vi "lerealtime.vi"() -> ()   [LabVIEW 2016]
uses:
  <vilib>/rvi/interface/nirviOpenFPGA/nirviOpenFPGA.xnode
  <vilib>/rvi/interface/nirviReadWriteControl/nirviReadWriteControl.xnode
  le fpga/le fpga.vi
  NiFpgaLv.dll
  <vilib>/Utility/error.llb/Error Cluster From Error Code.vi
  <vilib>/rvi/errors/niLvFpgaAdjustHostInterfaceError.vi
  FPGA Bitfiles/Controlsoftware2_FPGATarget2_lefpga_X2lKp2O+XjE.lvbitx
  <vilib>/FPGAPlugInAG/cRIO-9074/niLvFpga_Open_cRIO-9074.vi
panel:
  in  "Numeric value out":dbl
  in  "Tab Control":enum32{"Control", "Junk"}(tab)
  out "LE Einzel":dbl
  out "le waist einzel I":fxp<+/-,26,5> format="%.3g"
  out "le Waist Einzel V":fxp<+/-,26,5> format="%.3g"
  out "le waist Y-I":fxp<+/-,26,5> format="%.3g"
  out "le waist Y-V":fxp<+/-,26,5> format="%.3g"
  out "le waist Y+I":fxp<+/-,26,5> format="%.3g"
  out "le waist Y+ V":fxp<+/-,26,5> format="%.3g"
  out "le waist X-I":fxp<+/-,26,5> format="%.3g"
  out "le waist X- V":fxp<+/-,26,5> format="%.3g"
  out "le waist X+ I":fxp<+/-,26,5> format="%.3g"
  out "le waist X+ V":fxp<+/-,26,5> format="%.3g"
  out "le waist Y Steerer -":dbl
  out "le waist Y Steerer +":dbl
  out "le waistX Steerer -":dbl
  out "le waist X Steerer +":dbl
  out "Tank entrance Cryo pump":T1
  out "atten":bool
  out "LE waist fc":bool
  out "LE waist apt":bool
  out "inj image ap":bool
  out "tank entrance fc":bool
  out "Tank Entrance Ion gauge Cluster":T2
  out "LE Waist Ion gauge Cluster 2":T2
  out "Y Steerer -":dbl
  out "Y Steerer +":dbl
  out "X Steerer -":dbl
  out "X Steerer +":dbl
  out "Y Steerer -  2":dbl
  out "Y Steerer +  2":dbl
  in  "X Steerer - 2":dbl
  in  "X Steerer + 2":dbl
  out "Y-I 2":fxp<+/-,26,5> format="%.3g"
  out "Y-V 2":fxp<+/-,26,5> format="%.3g"
  out "Y+I 2":fxp<+/-,26,5> format="%.3g"
  out "Y+ V  2":fxp<+/-,26,5> format="%.3g"
  out "Y-I":fxp<+/-,26,5> format="%.3g"
  out "Y-V":fxp<+/-,26,5> format="%.3g"
  out "Y+I":fxp<+/-,26,5> format="%.3g"
  out "Y+ V":fxp<+/-,26,5> format="%.3g"
  out "X-I":fxp<+/-,26,5> format="%.3g"
  out "X- V":fxp<+/-,26,5> format="%.3g"
  out "X+ I":fxp<+/-,26,5> format="%.3g"
  out "X+ V":fxp<+/-,26,5> format="%.3g"
  out "X-I 2":fxp<+/-,26,5> format="%.3g"
  out "X- V  2":fxp<+/-,26,5> format="%.3g"
  out "X+ I 2":fxp<+/-,26,5> format="%.3g"
  out "X+ V 2":fxp<+/-,26,5> format="%.3g"
  out "Digital readback":bool[](array[boolean])
  out "inj cup fc":bool
  out "injector image fc in":bool
  out "injector image fc out":bool
  in  "Ion gauge cluster control":T2
  in  "Cryo pump 3":T3
  out "Convectron 2":u8[](array[numeric])
  out "Ion gauge 2":u8[](array[numeric])
  out "Convectron 1":u8[](array[numeric])
  out "Ion gauge 1":u8[](array[numeric])
  out "error out 5":errorcluster
  out "Analog input":fxp<+/-,26,5>[](array[numeric]) format="%.23g"
  out "Analog input 2":fxp<+/-,26,5>[](array[numeric]) format="%.23g"
  out "appended array":dbl[](array[numeric])
  # "DO mod 7\n0 inj image fc in\n1 inj image fc out\n2 tank entrance in\n3 tank entrance out\n4 atten in\n5 atten out\n6 le waist fc in\n7 le waist fc out\n8 inj image ap in\n9 inj image ap out"
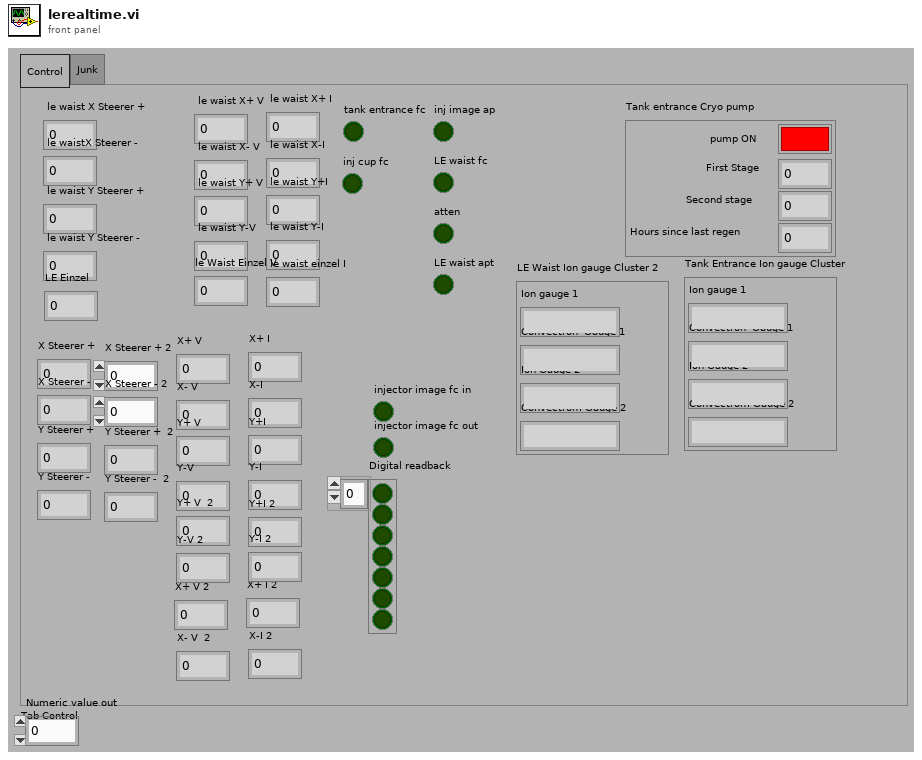
[diagram p1: front panel]
types:
  T1 = cluster{"First Stage":dbl, "Second stage":dbl, "Hours since last regen":dbl, "pump ON":bool}
  T2 = cluster{"Ion gauge 1":string, "Convectron  Gauge 1 ":string, "Ion Gauge 2":string, "Convectrom Gauge 2":string}
  T3 = cluster{"First Stage":dbl, "Second stage":dbl, "Hours since last regen":dbl, "Pump ON":bool}
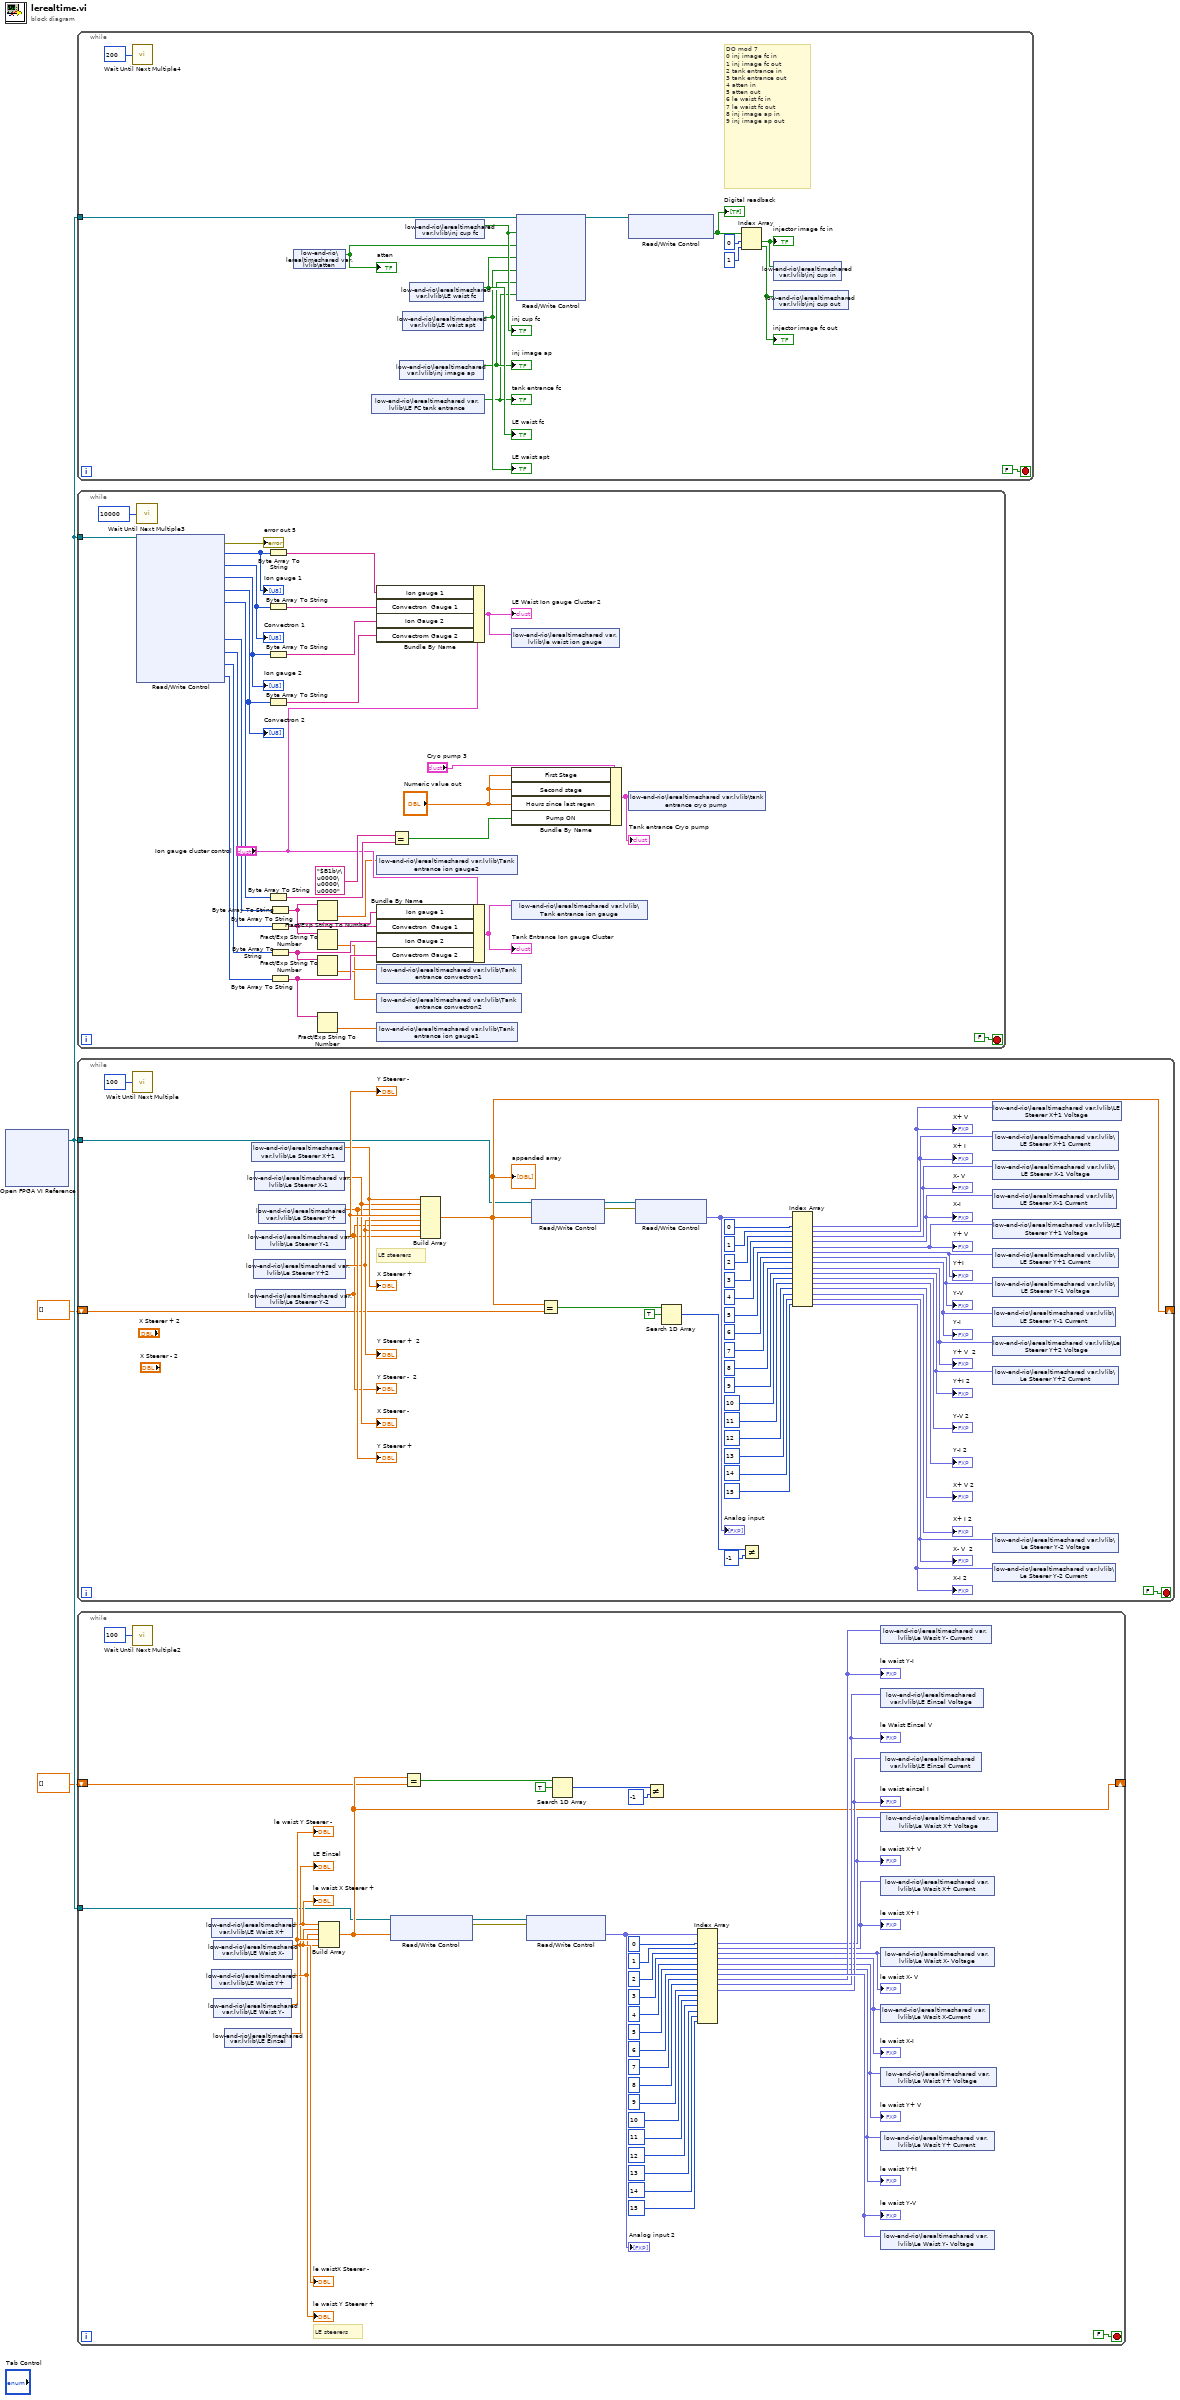
[diagram p0: block diagram]
diagram:
  n1 = xnode "Open FPGA VI Reference"() -> ("FPGA VI Reference Out"=w3:refnum<k20>)  [unwired: 2 in, 1 out]
  n2 = while {
    tunnel: w3 -> [w18]
    stop <- FALSE stop-if-true
    # "DO mod 7\n0 inj image fc in\n1 inj image fc out\n2 tank entrance in\n3 tank entrance out\n4 atten in\n5 atten out\n6 le waist fc in\n7 le waist fc out\n8 inj image ap in\n9 inj image ap out"
    n3 = call "Wait Until Next Multiple4"("Count(mSec)"=u32 200) -> ()  [unwired: 1 out]
    n4 = shared-variable "low-end-rio\\lerealtimeshared var.lvlib\\atten"() -> (w12:bool)  [unwired: 1 in, 1 out]
    "atten" <- w12
    n5 = shared-variable "low-end-rio\\lerealtimeshared var.lvlib\\LE FC tank entrance"() -> (w10:bool)  [unwired: 1 in, 1 out]
    "tank entrance fc" <- w10
    n6 = shared-variable "low-end-rio\\lerealtimeshared var.lvlib\\inj image ap"() -> (w13:bool)  [unwired: 1 in, 1 out]
    "inj image ap" <- w13
    n7 = shared-variable "low-end-rio\\lerealtimeshared var.lvlib\\LE waist apt"() -> (w14:bool)  [unwired: 1 in, 1 out]
    "LE waist apt" <- w14
    n8 = shared-variable "low-end-rio\\lerealtimeshared var.lvlib\\LE waist fc"() -> (w15:bool)  [unwired: 1 in, 1 out]
    "LE waist fc" <- w15
    n9 = shared-variable "low-end-rio\\lerealtimeshared var.lvlib\\inj cup fc"() -> (w17:bool)  [unwired: 1 in, 1 out]
    "inj cup fc" <- w17
    n10 = xnode "Read/Write Control"("FPGA VI Reference In"=w18, "inj image  FC"=w17, "ATTEN"=w12, "LE Waist FC"=w15, "LE waist ap"=w14, "inj image ap"=w13, "LE FC"=w10) -> ("FPGA VI Reference Out"=w11:refnum<k20>)  [unwired: 1 in, 1 out]
    n11 = xnode "Read/Write Control"("FPGA VI Reference In"=w11) -> ("Digital readback"=w9:bool[])  [unwired: 1 in, 2 out]
    "Digital readback" <- w9
    n12 = Index Array(array=w9, index #1=0 ("index"), index #2=1 ("index")) -> (element #1=w7:bool, element #2=w5:bool)
    "injector image fc in" <- w7
    "injector image fc out" <- w5
    n13 = shared-variable "low-end-rio\\lerealtimeshared var.lvlib\\inj cup in"(w7) -> ()  [unwired: 1 in, 1 out]
    n14 = shared-variable "low-end-rio\\lerealtimeshared var.lvlib\\inj cup out"(w5) -> ()  [unwired: 1 in, 1 out]
  }
  n15 = while {
    tunnel: w3 -> [w47]
    stop <- FALSE stop-if-true
    n16 = call "Wait Until Next Multiple3"("Count(mSec)"=u32 10000) -> ()  [unwired: 1 out]
    n17 = xnode "Read/Write Control"("FPGA VI Reference In"=w47) -> ("error out"=→"error out 5":errorcluster, "Ion gauge 3"=w46:u8[], "Convectron 3"=w45:u8[], "Convectron 4"=w44:u8[], "Ion gauge 4"=w43:u8[], "Pump On"=w37:u8[], "Ion gauge 5"=w27:u8[], "Convectron 5"=w35:u8[], "Convectron 6"=w34:u8[], "Ion gauge 6"=w33:u8[])  [unwired: 1 in, 3 out]
    "Ion gauge 1" <- w46
    "Convectron 1" <- w45
    "Ion gauge 2" <- w44
    "Convectron 2" <- w43
    n18 = Byte Array To String(unsigned byte array=w46) -> (string=w51:string)
    n19 = Byte Array To String(unsigned byte array=w45) -> (string=w50:string)
    n20 = Byte Array To String(unsigned byte array=w44) -> (string=w49:string)
    n21 = Byte Array To String(unsigned byte array=w43) -> (string=w48:string)
    n22 = Byte Array To String(unsigned byte array=w37) -> (string=w39:string)
    n23 = Byte Array To String(unsigned byte array=w27) -> (string=w26:string)
    n24 = Byte Array To String(unsigned byte array=w35) -> (string=w25:string)
    n25 = Byte Array To String(unsigned byte array=w34) -> (string=w24:string)
    n26 = Byte Array To String(unsigned byte array=w33) -> (string=w23:string)
    n27 = Fract/Exp String To Number(string=w26) -> (number=w20:dbl)  [unwired: 3 in, 1 out]
    n28 = Fract/Exp String To Number(string=w25) -> (number=w21:dbl)  [unwired: 3 in, 1 out]
    n29 = Fract/Exp String To Number(string=w24) -> (number=w22:dbl)  [unwired: 3 in, 1 out]
    n30 = Fract/Exp String To Number(string=w23) -> (number=w19:dbl)  [unwired: 3 in, 1 out]
    n31 = Bundle By Name(cluster="Ion gauge cluster control", "Ion gauge 1"=w51, "Convectron  Gauge 1"=w50, "Ion Gauge 2"=w49, "Convectrom Gauge 2"=w48) -> (w30:T2)
    "LE Waist Ion gauge Cluster 2" <- w30
    n32 = shared-variable "low-end-rio\\lerealtimeshared var.lvlib\\Tank entrance ion gauge2"(w20) -> ()  [unwired: 1 in, 1 out]
    n33 = Bundle By Name(cluster="Ion gauge cluster control", "Ion gauge 1"=w26, "Convectron  Gauge 1"=w25, "Ion Gauge 2"=w24, "Convectrom Gauge 2"=w23) -> (w29:T2)
    "Tank Entrance Ion gauge Cluster" <- w29
    n34 = shared-variable "low-end-rio\\lerealtimeshared var.lvlib\\Tank entrance convectron1"(w21) -> ()  [unwired: 1 in, 1 out]
    n35 = shared-variable "low-end-rio\\lerealtimeshared var.lvlib\\Tank entrance convectron2"(w22) -> ()  [unwired: 1 in, 1 out]
    n36 = shared-variable "low-end-rio\\lerealtimeshared var.lvlib\\Tank entrance ion gauge1"(w19) -> ()  [unwired: 1 in, 1 out]
    n37 = Equal?(x="$B1b\r\u0000\u0000\u0000" ("string 2"), y=w39) -> (x = y?=w36:bool)
    n38 = shared-variable "low-end-rio\\lerealtimeshared var.lvlib\\le waist ion gauge"(w30) -> ()  [unwired: 1 in, 1 out]
    n39 = Bundle By Name(cluster="Cryo pump 3", "First Stage"="Numeric value out", "Second stage"="Numeric value out", "Hours since last regen"="Numeric value out", "Pump ON"=w36) -> (w31:T3)
    "Tank entrance Cryo pump" <- w31
    n40 = shared-variable "low-end-rio\\lerealtimeshared var.lvlib\\Tank entrance ion gauge"(w29) -> ()  [unwired: 1 in, 1 out]
    n41 = shared-variable "low-end-rio\\lerealtimeshared var.lvlib\\tank entrance cryo pump"(w31) -> ()  [unwired: 1 in, 1 out]
  }
  n42 = while {
    tunnel: w3 -> [w53]
    shift-right: [w55] -> _
    shift-left: dbl[] [] -> [w56]
    stop <- FALSE stop-if-true
    # "LE steerers"
    n43 = call "Wait Until Next Multiple"("Count(mSec)"=u32 100) -> ()  [unwired: 1 out]
    n44 = shared-variable "low-end-rio\\lerealtimeshared var.lvlib\\Le Steerer X+1"() -> (w64:dbl)  [unwired: 1 in, 1 out]
    "X Steerer +" <- w64
    n45 = shared-variable "low-end-rio\\lerealtimeshared var.lvlib\\Le Steerer Y+2"() -> (w61:dbl)  [unwired: 1 in, 1 out]
    "Y Steerer +  2" <- w61
    n46 = shared-variable "low-end-rio\\lerealtimeshared var.lvlib\\Le Steerer X-1"() -> (w63:dbl)  [unwired: 1 in, 1 out]
    "X Steerer -" <- w63
    n47 = shared-variable "low-end-rio\\lerealtimeshared var.lvlib\\Le Steerer Y-1"() -> (w65:dbl)  [unwired: 1 in, 1 out]
    "Y Steerer -" <- w65
    n48 = shared-variable "low-end-rio\\lerealtimeshared var.lvlib\\Le Steerer Y-2"() -> (w60:dbl)  [unwired: 1 in, 1 out]
    "Y Steerer -  2" <- w60
    n49 = shared-variable "low-end-rio\\lerealtimeshared var.lvlib\\Le Steerer Y+"() -> (w62:dbl)  [unwired: 1 in, 1 out]
    "Y Steerer +" <- w62
    n50 = Build Array(w64, w63, w62, w65, w61, w60, w61, w60) -> (w55:dbl[])
    "appended array" <- w55
    n51 = xnode "Read/Write Control"("FPGA VI Reference In"=w53, "analog output"=w55) -> ("FPGA VI Reference Out"=w83:refnum<k20>, "error out"=w82:errorcluster)  [unwired: 1 in]
    n52 = Equal?(x=w55, y=w56) -> (x = y?=w57:bool[])
    n53 = xnode "Read/Write Control"("FPGA VI Reference In"=w83, "error in"=w82) -> ("Analog input"=w96:fxp<+/-,26,5>[])  [unwired: 2 out]
    "Analog input" <- w96
    n54 = Search 1D Array(1D array=w57, element=TRUE) -> (index of element=w58:i32)  [unwired: 1 in]
    n55 = Not Equal?(x=w58, y=-1) -> ()  [unwired: 1 out]
    n56 = Index Array(array=w96, index #1=0 ("index"), index #2=1 ("index"), index #3=2 ("index"), index #4=3 ("index"), index #5=4 ("index"), index #6=5 ("index"), index #7=6 ("index"), index #8=7 ("index"), index #9=8 ("index"), index #10=9 ("index"), index #11=10 ("index"), index #12=11 ("index"), index #13=12 ("index"), index #14=13 ("index"), index #15=14 ("index"), index #16=15 ("index")) -> (element #1=w67:fxp<+/-,26,5>, element #2=w66:fxp<+/-,26,5>, element #3=w69:fxp<+/-,26,5>, element #4=w68:fxp<+/-,26,5>, element #5=w71:fxp<+/-,26,5>, element #6=w70:fxp<+/-,26,5>, element #7=w75:fxp<+/-,26,5>, element #8=w74:fxp<+/-,26,5>, element #9=w73:fxp<+/-,26,5>, element #10=w72:fxp<+/-,26,5>, element #11=→"Y-V 2":fxp<+/-,26,5>, element #12=→"Y-I 2":fxp<+/-,26,5>, element #13=→"X+ V 2":fxp<+/-,26,5>, element #14=→"X+ I 2":fxp<+/-,26,5>, element #15=w77:fxp<+/-,26,5>, element #16=w76:fxp<+/-,26,5>)
    "X+ V" <- w67
    "X+ I" <- w66
    "X- V" <- w69
    "X-I" <- w68
    "Y+ V" <- w71
    "Y+I" <- w70
    "Y-V" <- w75
    "Y-I" <- w74
    "Y+ V  2" <- w73
    "Y+I 2" <- w72
    "X- V  2" <- w77
    "X-I 2" <- w76
    n57 = shared-variable "low-end-rio\\lerealtimeshared var.lvlib\\LE Steerer X+1 Voltage"(w67) -> ()  [unwired: 1 in, 1 out]
    n58 = shared-variable "low-end-rio\\lerealtimeshared var.lvlib\\LE Steerer X+1 Current"(w66) -> ()  [unwired: 1 in, 1 out]
    n59 = shared-variable "low-end-rio\\lerealtimeshared var.lvlib\\LE Steerer X-1 Voltage"(w69) -> ()  [unwired: 1 in, 1 out]
    n60 = shared-variable "low-end-rio\\lerealtimeshared var.lvlib\\LE Steerer X-1 Current"(w68) -> ()  [unwired: 1 in, 1 out]
    n61 = shared-variable "low-end-rio\\lerealtimeshared var.lvlib\\LE Steerer Y+1 Voltage"(w71) -> ()  [unwired: 1 in, 1 out]
    n62 = shared-variable "low-end-rio\\lerealtimeshared var.lvlib\\LE Steerer Y+1 Current"(w70) -> ()  [unwired: 1 in, 1 out]
    n63 = shared-variable "low-end-rio\\lerealtimeshared var.lvlib\\LE Steerer Y-1 Voltage"(w75) -> ()  [unwired: 1 in, 1 out]
    n64 = shared-variable "low-end-rio\\lerealtimeshared var.lvlib\\LE Steerer Y-1 Current"(w74) -> ()  [unwired: 1 in, 1 out]
    n65 = shared-variable "low-end-rio\\lerealtimeshared var.lvlib\\Le Steerer Y+2 Voltage"(w73) -> ()  [unwired: 1 in, 1 out]
    n66 = shared-variable "low-end-rio\\lerealtimeshared var.lvlib\\Le Steerer Y+2 Current"(w72) -> ()  [unwired: 1 in, 1 out]
    n67 = shared-variable "low-end-rio\\lerealtimeshared var.lvlib\\Le Steerer Y-2 Voltage"(w77) -> ()  [unwired: 1 in, 1 out]
    n68 = shared-variable "low-end-rio\\lerealtimeshared var.lvlib\\Le Steerer Y-2 Current"(w76) -> ()  [unwired: 1 in, 1 out]
  }
  n69 = while {
    tunnel: w3 -> [w103]
    shift-right: [w105] -> _
    shift-left: dbl[] [] -> [w104]
    stop <- FALSE stop-if-true
    # "LE steerers"
    n70 = call "Wait Until Next Multiple2"("Count(mSec)"=u32 100) -> ()  [unwired: 1 out]
    n71 = shared-variable "low-end-rio\\lerealtimeshared var.lvlib\\LE Waist X+"() -> (w113:dbl)  [unwired: 1 in, 1 out]
    "le waist X Steerer +" <- w113
    n72 = shared-variable "low-end-rio\\lerealtimeshared var.lvlib\\LE Waist Y+"() -> (w111:dbl)  [unwired: 1 in, 1 out]
    "le waist Y Steerer +" <- w111
    n73 = shared-variable "low-end-rio\\lerealtimeshared var.lvlib\\LE Waist X-"() -> (w112:dbl)  [unwired: 1 in, 1 out]
    "le waistX Steerer -" <- w112
    n74 = shared-variable "low-end-rio\\lerealtimeshared var.lvlib\\LE Waist Y-"() -> (w114:dbl)  [unwired: 1 in, 1 out]
    "le waist Y Steerer -" <- w114
    n75 = shared-variable "low-end-rio\\lerealtimeshared var.lvlib\\LE Einzel"() -> (w110:dbl)  [unwired: 1 in, 1 out]
    "LE Einzel" <- w110
    n76 = Build Array(w113, w112, w111, w114, w110) -> (w105:dbl[])
    n77 = xnode "Read/Write Control"("FPGA VI Reference In"=w103, "analog output 2"=w105) -> ("FPGA VI Reference Out"=w128:refnum<k20>, "error out"=w127:errorcluster)  [unwired: 1 in]
    n78 = Equal?(x=w105, y=w104) -> (x = y?=w109:bool[])
    n79 = xnode "Read/Write Control"("FPGA VI Reference In"=w128, "error in"=w127) -> ("Analog input  2"=w141:fxp<+/-,26,5>[])  [unwired: 2 out]
    "Analog input 2" <- w141
    n80 = Search 1D Array(1D array=w109, element=TRUE) -> (index of element=w107:i32)  [unwired: 1 in]
    n81 = Not Equal?(x=w107, y=-1) -> ()  [unwired: 1 out]
    n82 = Index Array(array=w141, index #1=0 ("index"), index #2=1 ("index"), index #3=2 ("index"), index #4=3 ("index"), index #5=4 ("index"), index #6=5 ("index"), index #7=6 ("index"), index #8=7 ("index"), index #9=8 ("index"), index #10=9 ("index"), index #11=10 ("index"), index #12=11 ("index"), index #13=12 ("index"), index #14=13 ("index"), index #15=14 ("index"), index #16=15 ("index")) -> (element #1=w116:fxp<+/-,26,5>, element #2=w115:fxp<+/-,26,5>, element #3=w118:fxp<+/-,26,5>, element #4=w117:fxp<+/-,26,5>, element #5=w120:fxp<+/-,26,5>, element #6=w119:fxp<+/-,26,5>, element #7=w124:fxp<+/-,26,5>, element #8=w123:fxp<+/-,26,5>, element #9=w122:fxp<+/-,26,5>, element #10=w121:fxp<+/-,26,5>)  [unwired: 6 out]
    "le waist X+ V" <- w116
    "le waist X+ I" <- w115
    "le waist X- V" <- w118
    "le waist X-I" <- w117
    "le waist Y+ V" <- w120
    "le waist Y+I" <- w119
    "le waist Y-V" <- w124
    "le waist Y-I" <- w123
    "le Waist Einzel V" <- w122
    "le waist einzel I" <- w121
    n83 = shared-variable "low-end-rio\\lerealtimeshared var.lvlib\\Le Wasit Y- Current"(w123) -> ()  [unwired: 1 in, 1 out]
    n84 = shared-variable "low-end-rio\\lerealtimeshared var.lvlib\\LE Einzel Voltage"(w122) -> ()  [unwired: 1 in, 1 out]
    n85 = shared-variable "low-end-rio\\lerealtimeshared var.lvlib\\LE Einzel Current"(w121) -> ()  [unwired: 1 in, 1 out]
    n86 = shared-variable "low-end-rio\\lerealtimeshared var.lvlib\\Le Waist X+ Voltage"(w116) -> ()  [unwired: 1 in, 1 out]
    n87 = shared-variable "low-end-rio\\lerealtimeshared var.lvlib\\Le Wasit X+ Current"(w115) -> ()  [unwired: 1 in, 1 out]
    n88 = shared-variable "low-end-rio\\lerealtimeshared var.lvlib\\Le Waist X- Voltage"(w118) -> ()  [unwired: 1 in, 1 out]
    n89 = shared-variable "low-end-rio\\lerealtimeshared var.lvlib\\Le Wasit X-Current"(w117) -> ()  [unwired: 1 in, 1 out]
    n90 = shared-variable "low-end-rio\\lerealtimeshared var.lvlib\\Le Waist Y+ Voltage"(w120) -> ()  [unwired: 1 in, 1 out]
    n91 = shared-variable "low-end-rio\\lerealtimeshared var.lvlib\\Le Wasit Y+ Current"(w119) -> ()  [unwired: 1 in, 1 out]
    n92 = shared-variable "low-end-rio\\lerealtimeshared var.lvlib\\Le Waist Y- Voltage"(w124) -> ()  [unwired: 1 in, 1 out]
  }
